vi "ImpulseData - Get Saccade Stimulus Onset.vi"(0 "Saccade in":T1, 3 "error in (no error)":errorcluster, 4 "Impulse Data":refnum<data-value>) -> (7 "Saccade out":T1, 8 "Onset (idx)":dbl, 9 "Peak (idx)":dbl, 10 "error out":errorcluster)   [LabVIEW 2016]
uses:
  Type Definitions/Saccade Analyser Saccade Data.ctl
  Type Definitions/Saccade Analyser Impulse Data.ctl
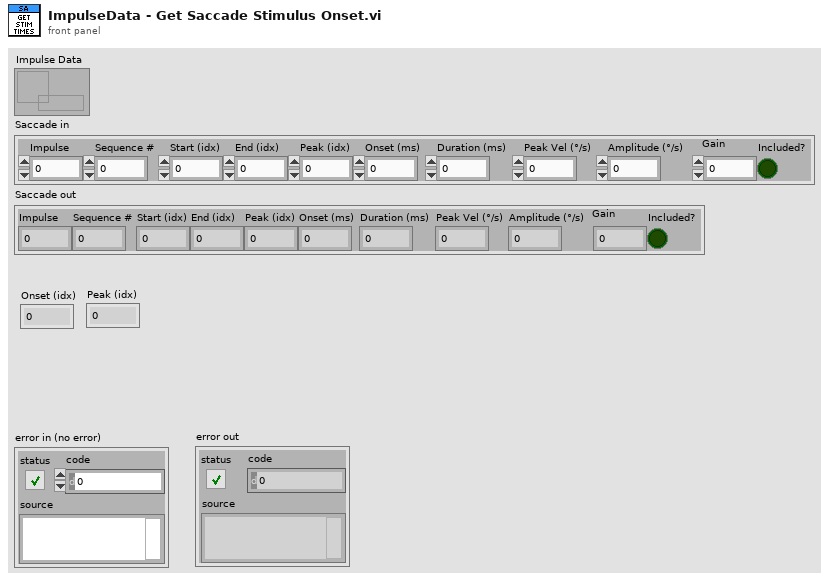
[diagram p1: front panel]
types:
  T1 = typedef "Saccade Analyser Saccade Data.ctl" = cluster{"Impulse":i32, "Sequence #":dbl, "Start (idx)":dbl, "End (idx)":dbl, "Peak (idx)":dbl, "Onset (ms)":dbl, "Duration (ms)":dbl, "Peak Vel (°/s)":dbl, "Amplitude (°/s)":dbl, "Gain":dbl, "Included?":bool}
  T2 = typedef "Saccade Analyser Impulse Data.ctl" = cluster{"Stimulus Data":dbl[], "Response Data":dbl[], "Peak (idx)":i32, "Onset (idx)":i32}
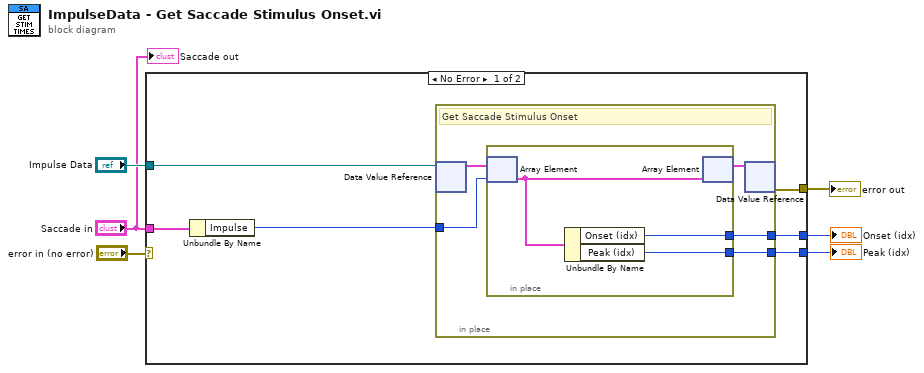
[diagram p0: block diagram]
diagram:
  n1 = case shown="No Error" "error in (no error)" {
    selector: "error in (no error)" -> [_ w21]
    tunnel: "Impulse Data" -> [w12 _]
    tunnel: "Saccade in" -> [w11 _]
    tunnel: [w9 w21] -> w3
    tunnel: [w8 _] -> w2
    tunnel: [w7 _] -> w1
    frame No Error {
      n2 = Unbundle By Name(w11) -> ("Impulse"=w10:i32)
      n3 = in-place {
        in-place-border: w10 -> [w15]
        in-place-border: [w14] -> w8
        in-place-border: [w13] -> w7
        # "Get Saccade Stimulus Onset"
        n4 = in-place-dvr #1(w12) -> (w17:T2[])  [unwired: 1 out]
        n5 = in-place {
          in-place-border: [w19] -> w14
          in-place-border: [w18] -> w13
          n6 = in-place-array #2(w17, w15) -> (w20:T2)
          n7 = Unbundle By Name(w20) -> ("Onset (idx)"=w19:i32, "Peak (idx)"=w18:i32)
          n8 = in-place-array #2(w20) -> (w16:T2[])  [unwired: 1 out]
        }
        n9 = in-place-dvr #1(w16) -> (w9:errorcluster)  [unwired: 1 out]
      }
    }
    frame Error {
    }
  }
  "error out" <- w3
  "Onset (idx)" <- w2
  "Peak (idx)" <- w1
  "Saccade out" <- "Saccade in"
